vi "LAC Cmd082_Ether Setting.vi"(6 "R/W (F:Read)":bool, 7 "timeout(ms)":u32=500, 8 "error in":errorcluster, 9 "NetSetting":T1={"IP_Addr"="192.168.0.100", "Subnet_Mask"="255.255.255.0", "Gateway"="0.0.0.0", "Port"="8000"}, 11 "VISA name in":refnum<visa-resource-name>) -> (0 "error out":errorcluster, 1 "readout":string, 3 "VISA name out":refnum<visa-resource-name>)   [LabVIEW 2018]
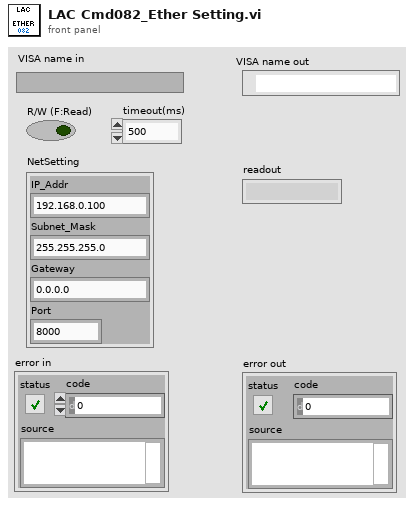
[diagram p1: front panel]
types:
  T1 = cluster{"IP_Addr":string, "Subnet_Mask":string, "Gateway":string, "Port":string}
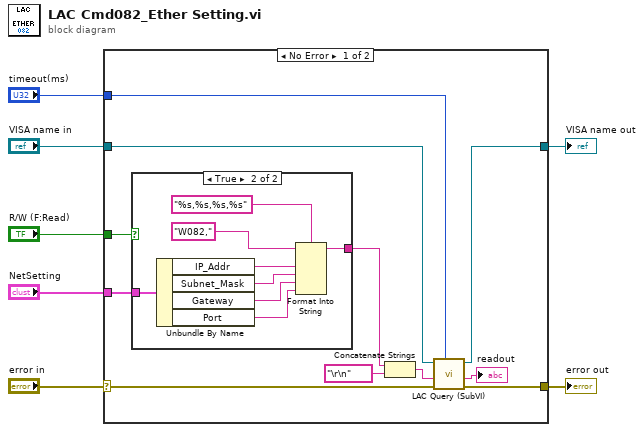
[diagram p0: block diagram]
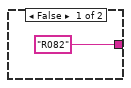
[diagram p2: hidden frame]
diagram:
  n1 = case shown="No Error" "error in" {
    selector: "error in" -> [w14 w29]
    tunnel: "VISA name in" -> [w16 w28]
    tunnel: [w18 w28] -> w6
    tunnel: [w17 w29] -> w5
    tunnel: "timeout(ms)" -> [w15 _]
    tunnel: "R/W (F:Read)" -> [w9 _]
    tunnel: "NetSetting" -> [w8 _]
    frame No Error {
      n2 = case shown="True" w9 {
        tunnel: ["R082" ("string") w25] -> w10
        tunnel: w8 -> [_ w24]
        frame False {
        }
        frame True {
          n3 = Unbundle By Name(w24) -> ("IP_Addr"=w23:string, "Subnet_Mask"=w22:string, "Gateway"=w21:string, "Port"=w20:string)
          n4 = Format Into String(format string="%s,%s,%s,%s", initial string="W082," ("string"), w23, w22, w21, w20) -> (resulting string=w25:string)  [unwired: 1 in, 1 out]
        }
      }
      n5 = Concatenate Strings(w10, "\r\n" ("write buffer")) -> (w12:string)
      n6 = call "LAC Query (SubVI).vi"("timeout(ms)"=w15, "error in"=w14, "Command"=w12, "VISA name in"=w16) -> ("error out"=w17:errorcluster, "read buffer"=→"readout":string, "VISA name out"=w18:refnum<visa-resource-name>)  [unwired: 5 in]
    }
    frame Error {
    }
  }
  "VISA name out" <- w6
  "error out" <- w5
